vi "CalculatePhaseSensitivity.vi"(2 "epsilon":dbl, 3 "n":i32, 4 "L":dbl) -> (1 "Czułość fazowa":dbl)   [LabVIEW 2015]
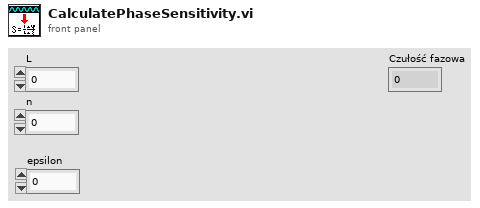
[diagram p1: front panel]
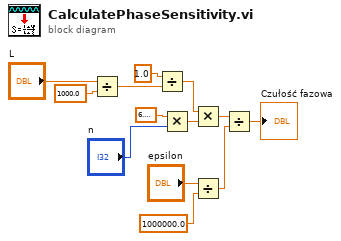
[diagram p0: block diagram]
diagram:
  n1 = Divide(x="L", y=1000.0) -> (x/y=w2:dbl)
  n2 = Divide(x=1.0, y=w2) -> (x/y=w3:dbl)
  n3 = Multiply(x=6.283185307179586, y="n") -> (x*y=w10:dbl)
  n4 = Multiply(x=w3, y=w10) -> (x*y=w9:dbl)
  n5 = Divide(x="epsilon", y=1000000.0) -> (x/y=w4:dbl)
  n6 = Divide(x=w9, y=w4) -> (x/y=→"Czułość fazowa":dbl)
